vi "CCD Acquire Spectrum.vi"(11 "error in":errorcluster) -> (15 "error out":errorcluster)   [LabVIEW 2023, in "Examples.lvlib"]
doc: "Example for a CCD spectrum acquisition."
uses:
  Classes/CCD/acquisitionImageData.ctl
  Classes/CCD/imageAcqData.ctl
  4aef6941-9f58-45d1-a797-2b486d7897ac.vi
  Classes/CCD/CCD.lvclass
  Examples.lvlib
panel:
  out "imageAcquisitions":T1[](array[typedef])
  # "Connector Pane"
  # "Locals"
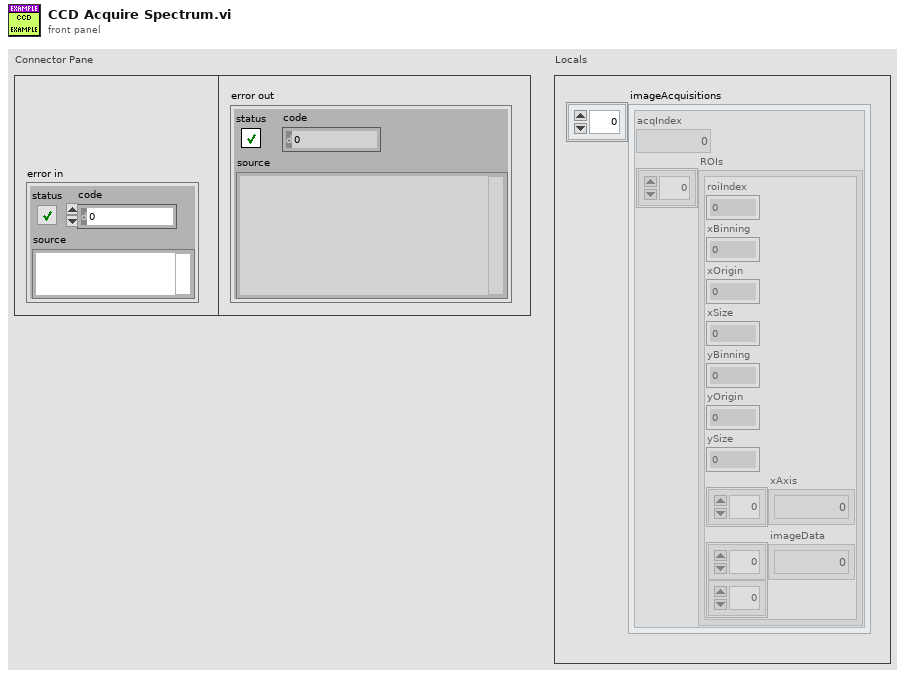
[diagram p1: front panel]
types:
  T1 = typedef "horiba.lvlib/CCD.lvclass/acquisitionImageData.ctl" = cluster{"acqIndex":i32, "ROIs":T2[]}
  T2 = typedef "horiba.lvlib/CCD.lvclass/imageAcqData.ctl" = cluster{"roiIndex":i32, "xBinning":i32, "xOrigin":i32, "xSize":i32, "yBinning":i32, "yOrigin":i32, "ySize":i32, "xAxis":dbl[], "imageData":dbl[][]}
  T3 = cluster{"ROI-index":i32, "xOrigin":i32, "yOrigin":i32, "xSize":i32, "ySize":i32, "xBin":i32, "yBin":i32}
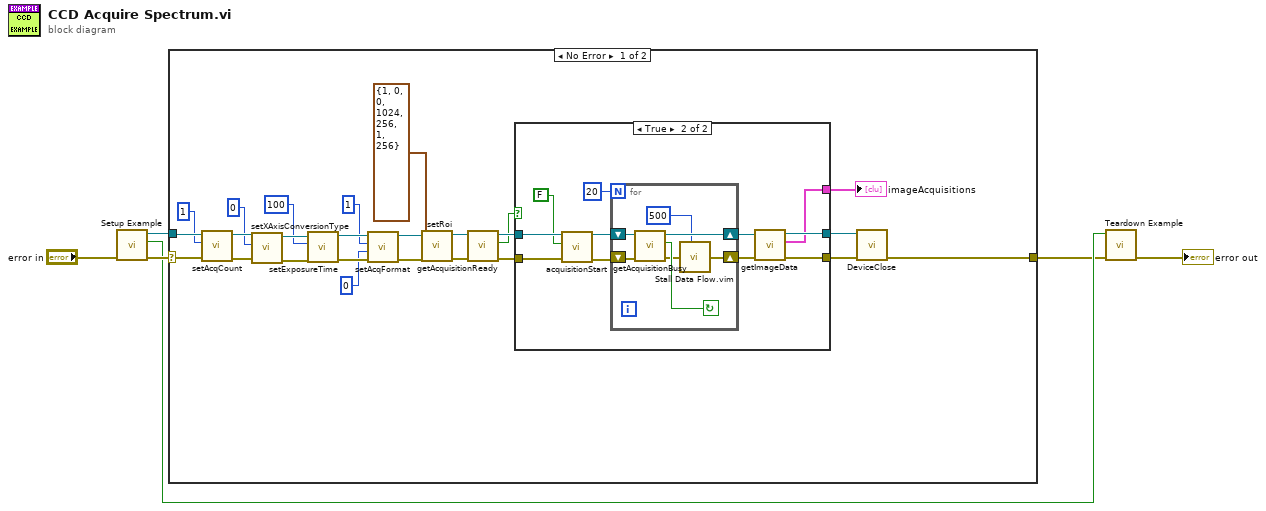
[diagram p0: block diagram]
diagram:
  n1 = call "Setup Example.vi"("error in (no error)"="error in") -> ("error out"=w4:errorcluster, "Module Was Already Running?"=w2:bool, "CCD out"=w3:refnum<class "CCD.lvclass">)  [unwired: 8 in]
  n2 = case shown="No Error" w4 {
    selector: w4 -> [w31 w52]
    tunnel: w3 -> [w30 _]
    tunnel: [w10 w52] -> w1
    frame No Error {
      n3 = call "setAcqCount.vi"("error in (no error)"=w31, "count"=1, "CCD in"=w30) -> ("error out"=w28:errorcluster, "CCD out"=w27:refnum<class "CCD.lvclass">)  [unwired: 5 in, 2 out]
      n4 = call "setXAxisConversionType.vi"("error in (no error)"=w28, "type"=0, "CCD in"=w27) -> ("error out"=w25:errorcluster, "CCD out"=w24:refnum<class "CCD.lvclass">)  [unwired: 5 in, 2 out]
      n5 = call "setExposureTime.vi"("error in (no error)"=w25, "exposure time [ms] or [us]"=100, "CCD in"=w24) -> ("error out"=w22:errorcluster, "CCD out"=w21:refnum<class "CCD.lvclass">)  [unwired: 5 in, 2 out]
      n6 = call "setAcqFormat.vi"("error in (no error)"=w22, "format"=0, "number of ROIs"=1, "CCD in"=w21) -> ("error out"=w18:errorcluster, "CCD out"=w17:refnum<class "CCD.lvclass">)  [unwired: 4 in, 2 out]
      n7 = call "setRoi.vi"("error in (no error)"=w18, "roiConfig"=T3 {"ROI-index"=1, "xOrigin"=0, "yOrigin"=0, "xSize"=1024, "ySize"=256, "xBin"=1, "yBin"=256}, "CCD in"=w17) -> ("error out"=w16:errorcluster, "CCD out"=w15:refnum<class "CCD.lvclass">)  [unwired: 5 in, 2 out]
      n8 = call "getAcquisitionReady.vi"("error in (no error)"=w16, "CCD in"=w15) -> ("error out"=w14:errorcluster, "ready"=w12:bool, "CCD out"=w13:refnum<class "CCD.lvclass">)  [unwired: 7 in]
      n9 = case shown="True" w12 {
        tunnel: w14 -> [w32 w44]
        tunnel: w13 -> [w33 w43]
        tunnel: [w32 w37] -> w11
        tunnel: [w33 w35] -> w9
        tunnel: [_ w34] -> w8
        frame False {
        }
        frame True {
          n10 = call "acquisitionStart.vi"("error in (no error)"=w44, "openShutter"=FALSE, "CCD in"=w43) -> ("error out"=w39:errorcluster, "CCD out"=w38:refnum<class "CCD.lvclass">)  [unwired: 5 in, 2 out]
          n11 = for {
            N: 20 -> [_]
            shift-right: [w47] -> w40
            shift-left: w39 -> [w50]
            shift-right: [w46] -> w36
            shift-left: w38 -> [w51]
            stop <- w49 continue-if-true
            n12 = call "getAcquisitionBusy.vi"("error in (no error)"=w50, "CCD in"=w51) -> ("error out"=w48:errorcluster, "isBusy"=w49:bool, "CCD out"=w46:refnum<class "CCD.lvclass">)  [unwired: 7 in]
            n13 = call "Stall Data Flow.vim"("value in"=w48, "milliseconds to wait"=u32 500) -> ("value out"=w47:errorcluster)  [unwired: 1 out]
          }
          n14 = call "getImageData.vi"("error in (no error)"=w40, "CCD in"=w36) -> ("error out"=w37:errorcluster, "imageAcquisitions"=w34:T1[], "CCD out"=w35:refnum<class "CCD.lvclass">)  [unwired: 6 in, 1 out]
        }
      }
      "imageAcquisitions" <- w8
      n15 = call-dynamic "DeviceClose.vi"("error in (no error)"=w11, "CCD in"=w9) -> ("error out"=w10:errorcluster)  [unwired: 5 in, 4 out]
    }
    frame Error {
    }
  }
  n16 = call "Teardown Example.vi"("error in (no error)"=w1, "Module Was Already Running?"=w2) -> ("error out"=→"error out":errorcluster)  [unwired: 9 in]
